vi "Scramble.vi"(0 "appended path":path, 1 "iw_data":dbl[][](array[numeric]), 5 "prb_num":dbl, 6 "UL_subframe_num":dbl, 7 "C":dbl, 9 "Qm":dbl, 11 "error in (no error)":errorcluster caption="错误输入（无错误）", 12 "ue_index":dbl, 13 "rm_len":dbl, 15 "cellid":dbl) -> (4 "scramble_data":dbl[](array[numeric]), 10 "error out":errorcluster caption="错误输出")   [LabVIEW 2015]
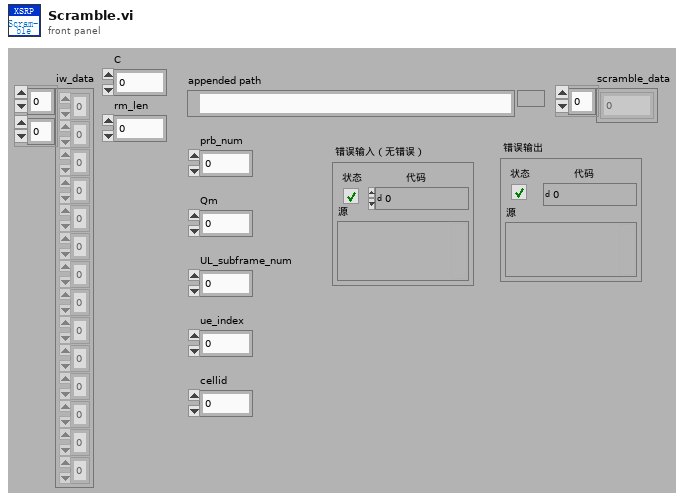
[diagram p1: front panel]
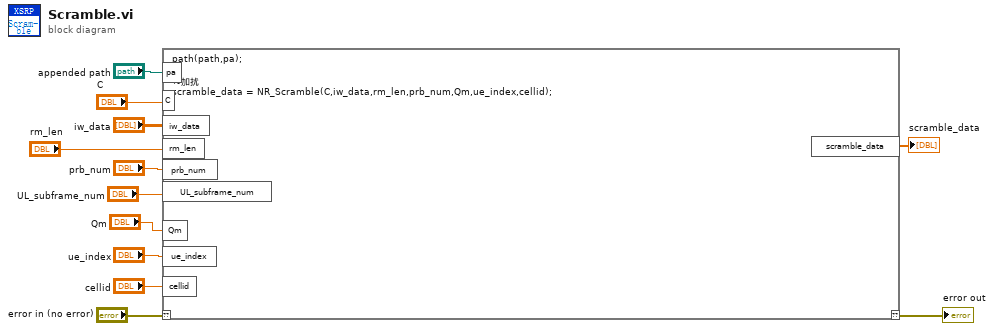
[diagram p0: block diagram]
diagram:
  n1 = script code="path(path,pa);\n\n%加扰\nscramble_data = NR_Scramble(C,iw_data,rm_len,prb_num,Qm,ue_index,cellid);"("??"="error in (no error)", "pa"="appended path", "iw_data"="iw_data", "prb_num"="prb_num", "Qm"="Qm", "UL_subframe_num"="UL_subframe_num", "ue_index"="ue_index", "cellid"="cellid", "C"="C", "rm_len"="rm_len") -> ("??"=→"error out":errorcluster, "scramble_data"=→"scramble_data":dbl[])
